vi "tcp_server.vi"() -> ()   [LabVIEW 2019]
panel:
  out "server_status_2":string
  out "error out 2":errorcluster
  out "server_step_2":i32
  in  "stop_server_2":bool
  out "error out":errorcluster
  out "EOS":bool=TRUE
  out "BOS":bool=TRUE
  out "server_step":i32
  out "spill_id":i32
  in  "stop_server":bool
  in  "stop_spill_inc":bool
  # "Spill-ID Inc."
  # "TCP/IP Server: ASAP Mode"
  # "TCP/IP Server: BOS Mode"
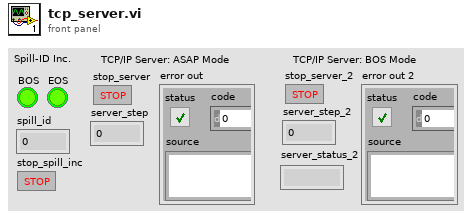
[diagram p1: front panel]
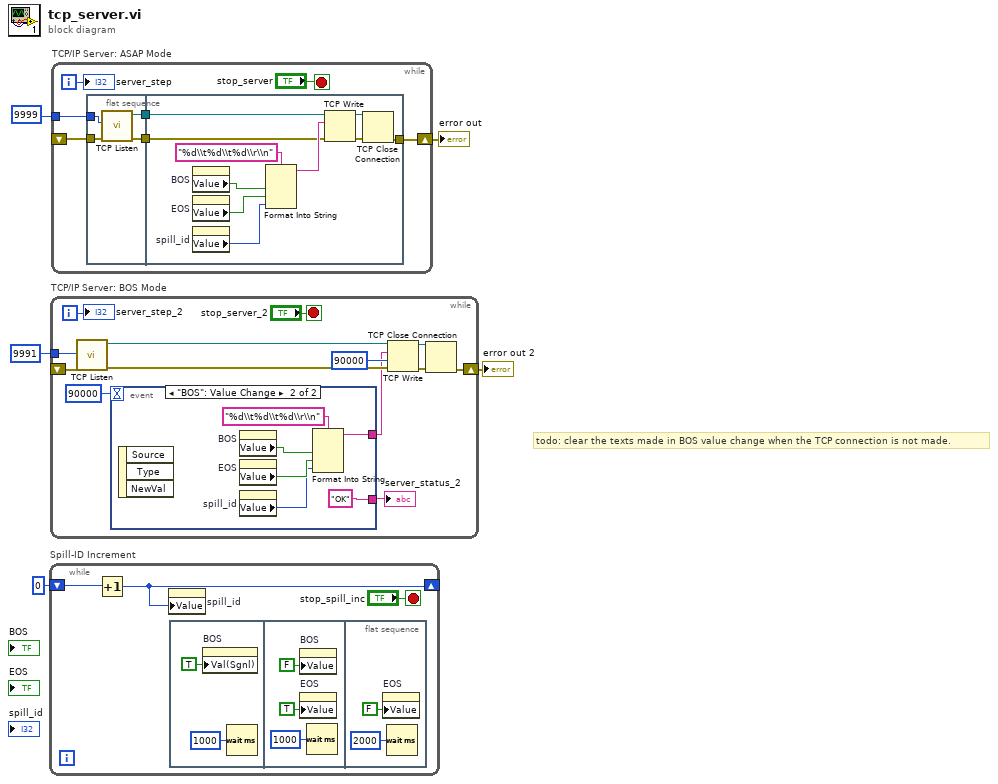
[diagram p0: block diagram]
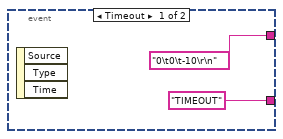
[diagram p2: hidden frame]
diagram:
  # "todo: clear the texts made in BOS value change when the TCP connection is not made."
  n1 = while "Spill-ID Increment" {
    shift-right: [w6] -> _
    shift-left: 0 -> [w8]
    stop <- "stop_spill_inc" stop-if-true
    n2 = Increment(x=w8) -> (x+1=w6:i32)
    n3 = property on="spill_id" class="DigNum (strict)"("Value"=w6) -> ()  [unwired: 2 in, 2 out]
    n4 = flat-sequence {
      frame #0 {
        n5 = property on="BOS" class="Bool (strict)"("Val(Sgnl)"=TRUE) -> ()  [unwired: 2 in, 2 out]
        n6 = Wait (ms)(milliseconds to wait=u32 1000) -> ()  [unwired: 1 out]
      }
      frame #1 {
        n7 = property on="BOS" class="Bool (strict)"("Value"=FALSE) -> ()  [unwired: 2 in, 2 out]
        n8 = property on="EOS" class="Bool (strict)"("Value"=TRUE) -> ()  [unwired: 2 in, 2 out]
        n9 = Wait (ms)(milliseconds to wait=u32 1000) -> ()  [unwired: 1 out]
      }
      frame #2 {
        n10 = property on="EOS" class="Bool (strict)"("Value"=FALSE) -> ()  [unwired: 2 in, 2 out]
        n11 = Wait (ms)(milliseconds to wait=u32 2000) -> ()  [unwired: 1 out]
      }
    }
  }
  n12 = while "TCP/IP Server: BOS Mode" {
    tunnel: u16 9991 ("port") -> [w23]
    shift-right: [w20] -> w2
    shift-left: _ -> [w19]
    i -> [w16]
    stop <- "stop_server_2" stop-if-true
    n13 = call <vilib>:"TCP Listen.vi"("error in (no error)"=w19, "port"=w23) -> ("error out"=w24:errorcluster, "connection ID"=w25:refnum<k5>)  [unwired: 5 in, 3 out]
    n14 = event shown="[1] \"BOS\": Value Change" {
      selector: _ -> [_ _]
      dyn-events: _ -> [_ _]
      timeout: 90000 -> [_ _]
      tunnel: ["0\t0\t-10\r\n" w36] -> w18
      tunnel: ["TIMEOUT" "OK"] -> w17
      event Timeout {
        n15 = event-data() -> ()  [unwired: 1 in, 3 out]
      }
      event "BOS": Value Change {
        n16 = event-data() -> ()  [unwired: 1 in, 3 out]
        n17 = property on="BOS" class="Bool (strict)"() -> ("Value"=w34:bool)  [unwired: 2 in, 2 out]
        n18 = property on="EOS" class="Bool (strict)"() -> ("Value"=w33:bool)  [unwired: 2 in, 2 out]
        n19 = property on="spill_id" class="DigNum (strict)"() -> ("Value"=w32:i32)  [unwired: 2 in, 2 out]
        n20 = Format Into String(format string="%d\\t%d\\t%d\\r\\n", w34, w33, w32) -> (resulting string=w36:string)  [unwired: 2 in, 1 out]
      }
    }
    "server_status_2" <- w17
    n21 = TCP Write(connection ID=w25, data in=w18, error in (no error)=w24, 9:90000 ("timeout ms (25000)")) -> (connection ID out=w26:refnum<k5>, error out=w27:errorcluster)  [unwired: 1 out]
    n22 = TCP Close Connection(connection ID=w26, error in (no error)=w27) -> (error out=w20:errorcluster)  [unwired: 1 in, 1 out]
    "server_step_2" <- w16
  }
  "error out 2" <- w2
  n23 = while "TCP/IP Server: ASAP Mode" {
    shift-right: [w42] -> w4
    shift-left: _ -> [w41]
    tunnel: u16 9999 ("port") -> [w40]
    i -> [w37]
    stop <- "stop_server" stop-if-true
    n24 = flat-sequence {
      tunnel: w40 -> [w44]
      tunnel: w41 -> [w47]
      tunnel: [w46] -> w39
      tunnel: [w45] -> w38
      tunnel: [w55] -> w42
      tunnel: w39 -> [w49]
      tunnel: w38 -> [w48]
      frame #0 {
        n25 = call <vilib>:"TCP Listen.vi"("error in (no error)"=w47, "port"=w44) -> ("error out"=w45:errorcluster, "connection ID"=w46:refnum<k5>)  [unwired: 5 in, 3 out]
      }
      frame #1 {
        n26 = property on="BOS" class="Bool (strict)"() -> ("Value"=w53:bool)  [unwired: 2 in, 2 out]
        n27 = property on="EOS" class="Bool (strict)"() -> ("Value"=w52:bool)  [unwired: 2 in, 2 out]
        n28 = property on="spill_id" class="DigNum (strict)"() -> ("Value"=w51:i32)  [unwired: 2 in, 2 out]
        n29 = Format Into String(format string="%d\\t%d\\t%d\\r\\n", w53, w52, w51) -> (resulting string=w50:string)  [unwired: 2 in, 1 out]
        n30 = TCP Write(connection ID=w49, data in=w50, error in (no error)=w48) -> (connection ID out=w56:refnum<k5>, error out=w57:errorcluster)  [unwired: 1 in, 1 out]
        n31 = TCP Close Connection(connection ID=w56, error in (no error)=w57) -> (error out=w55:errorcluster)  [unwired: 1 in, 1 out]
      }
    }
    "server_step" <- w37
  }
  "error out" <- w4
